vi "Log Data.vi"(8 "error in (no error)":errorcluster, 11 "MFC in":refnum<class "Valve.lvclass">) -> (0 "error out":errorcluster, 3 "MFC out":refnum<class "Valve.lvclass">)   [LabVIEW 2013, in "Valve.lvlib" / "Valve.lvclass"]
uses:
  Valve.lvclass
  Valve.lvclass/Valve.ctl
  Read Valve Position.vi
  PluginInterface/PluginInterface.lvlibp/PluginInterfaceClass/Read TDMS.vi
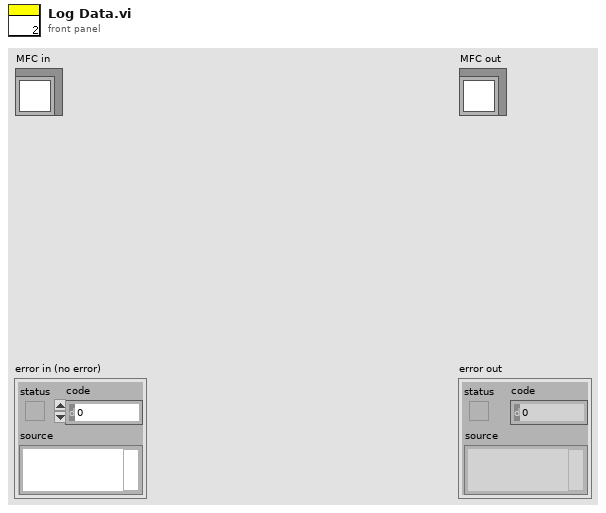
[diagram p1: front panel]
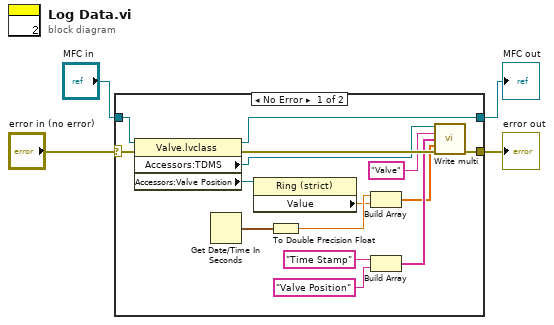
[diagram p0: block diagram]
diagram:
  n1 = case shown="No Error" "error in (no error)" {
    selector: "error in (no error)" -> [w9 w21]
    tunnel: [w8 w21] -> w3
    tunnel: [w17 w20] -> w1
    tunnel: "MFC in" -> [w18 w20]
    frame No Error {
      n2 = property class="Valve.lvclass"(reference=w18, error in=w9) -> (reference out=w17:refnum<class "Valve.lvclass">, error out=w16:errorcluster, "Accessors:TDMS"=w15:refnum<k34>, "Accessors:Valve Position"=w7:refnum<vi>)
      n3 = Get Date/Time In Seconds() -> (seconds since 1Jan1904=w19:timestamp)
      n4 = property class="Ring (strict)"(reference=w7) -> ("Value"=w6:dbl)  [unwired: 1 in, 2 out]
      n5 = To Double Precision Float(number=w19) -> (double precision float=w10:dbl)
      n6 = Build Array(w10, w6) -> (w5:dbl[])
      n7 = Build Array("Time Stamp" ("Channel"), "Valve Position" ("string")) -> (w11:string[])
      n8 = call "Write multi.vi"("tdms file in"=w15, "group"="Valve", "Channel"=w11, "Data"=w5, "error in (no error)"=w16) -> ("error out"=w8:errorcluster)  [unwired: 7 in, 3 out]
    }
    frame Error {
    }
  }
  "error out" <- w3
  "MFC out" <- w1
